vi "BotspeakSettingsUsed.vi"() -> ()   [LabVIEW 2014]
uses:
  <userlib>/BotSpeak/VIs/Direct/BotSpeak_Control.ctl
panel:
  in  "Bot Settings":T1
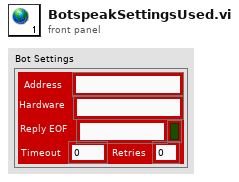
[diagram p1: front panel]
types:
  T1 = typedef "BotSpeak_Control.ctl" = cluster{"Address":string, "Reply EOF":string, "Hardware":string, "Retries":i8, "Timeout":i32, "Open?":bool}
diagram:
